vi "main.vi"() -> ()   [LabVIEW 2023]
panel:
  out "data out":string
  in  "Port":u16=12345
  out "Waveform Chart":dbl(graph)=0.0634239196565645
  in  "stop":bool
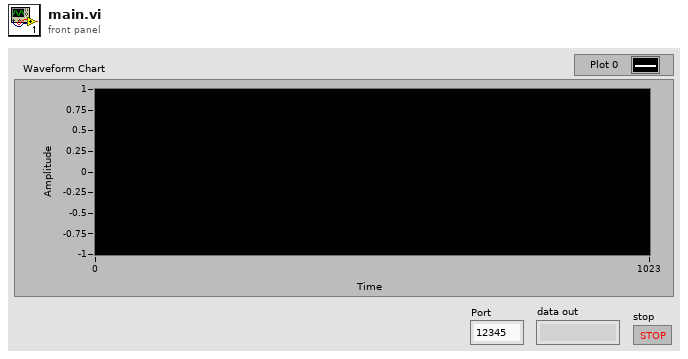
[diagram p1: front panel]
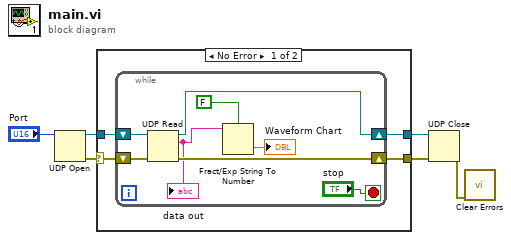
[diagram p0: block diagram]
diagram:
  n1 = UDP Open(11:"Port") -> (port=w4:refnum<k16>, 0:w3:errorcluster)  [unwired: 4 in, 1 out]
  n2 = case shown="No Error" w3 {
    selector: w3 -> [w7 w19]
    tunnel: [w10 w20] -> w6
    tunnel: [w9 w19] -> w5
    tunnel: w4 -> [w8 w20]
    frame No Error {
      n3 = while {
        shift-right: [w17] -> w10
        shift-left: w8 -> [w18]
        shift-right: [w15] -> w9
        shift-left: w7 -> [w16]
        stop <- "stop" stop-if-true
        n4 = UDP Read(connection ID=w18, 8:w16) -> (data out=w13:string, error out=w15:errorcluster, 3:w17:refnum<k16>)  [unwired: 2 in, 2 out]
        "data out" <- w13
        n5 = Fract/Exp String To Number(use system decimal point (T)=FALSE, string=w13) -> (number=→"Waveform Chart":dbl)  [unwired: 2 in, 1 out]
      }
    }
    frame Error {
    }
  }
  n6 = UDP Close(connection ID=w6, 8:w5) -> (error out=w1:errorcluster)  [unwired: 1 out]
  n7 = call <vilib>:"Clear Errors.vi"("error in (no error)"=w1) -> ()  [unwired: 5 in, 2 out]
